vi "Send and Receive Message.vi"(4 "timeout (ms) [100]":i32=100, 6 "Wait for response [T]":bool=TRUE, 8 "error in (no error)":errorcluster, 9 "Data":variant, 10 "Command":string, 11 "RemoteControl in":refnum<class "RemoteControl.lvclass">) -> (0 "error out":errorcluster, 1 "Data out":variant, 2 "Command out":string, 3 "RemoteControl out":refnum<class "RemoteControl.lvclass">)   [LabVIEW 2019, in "RemoteControl.lvclass"]
uses:
  RemoteControl.lvclass
  <userlib>/_OpenG.lib/numeric/numeric.llb/Random Number Within Range - I32__ogtk.vi
  <vilib>/Utility/error.llb/Error Cluster From Error Code.vi
  <vilib>/ErrorRing/Error Ring.xnode
panel:
  out "Numeric":i32
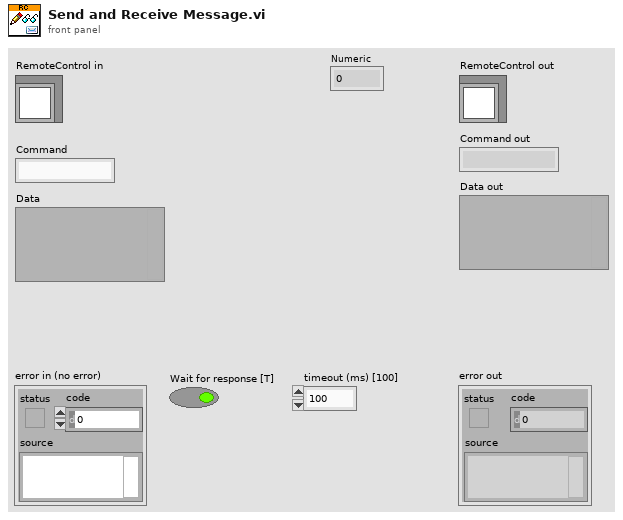
[diagram p1: front panel]
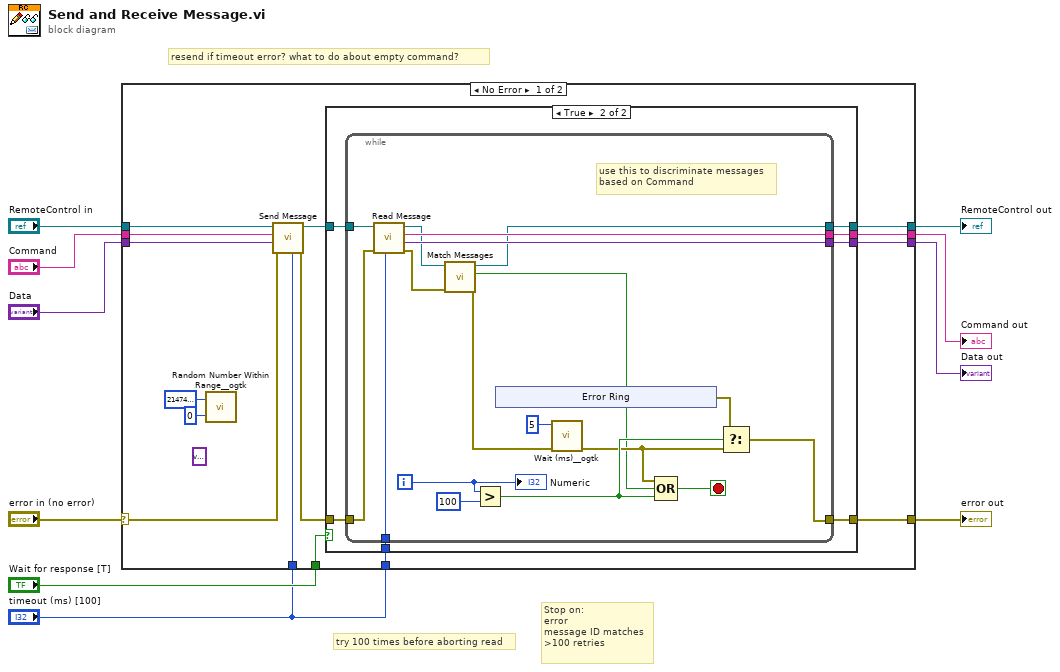
[diagram p0: block diagram]
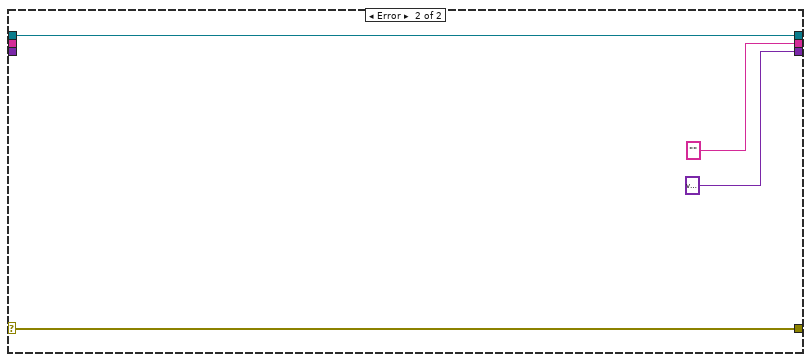
[diagram p3: hidden frame]
diagram:
  # "Stop on:\nerror\nmessage ID matches\n>100 retries"
  # "resend if timeout error? what to do about empty command?"
  # "try 100 times before aborting read"
  n1 = case shown="No Error" "error in (no error)" {
    selector: "error in (no error)" -> [w13 w60]
    tunnel: [w14 w60] -> w9
    tunnel: [w20 w59] -> w7
    tunnel: "RemoteControl in" -> [w22 w59]
    tunnel: "Wait for response [T]" -> [w25 _]
    tunnel: "timeout (ms) [100]" -> [w24 _]
    tunnel: "timeout (ms) [100]" -> [w21 _]
    tunnel: "Command" -> [w11 _]
    tunnel: "Data" -> [w19 _]
    tunnel: [w18 "" ("Command")] -> w2
    tunnel: [w17 variant ("Data")] -> w1
    frame No Error {
      (unwired) variant
      n2 = call-poly <userlib>:"Random Number Within Range__ogtk.vi"("High"=2147483647, "Low"=0) -> ()  [unwired: 3 in, 1 out]
      n3 = call-dynamic "Send Message.vi"("timeout in ms (100)"=w21, "error in (no error)"=w13, "Data"=w19, "Command"=w11, "RemoteControl in"=w22) -> ("error out"=w12:errorcluster, "RemoteControl out"=w23:refnum<class "RemoteControl.lvclass">)  [unwired: 4 in, 1 out]
      n4 = case shown="True" w25 {
        tunnel: w23 -> [w26 w34]
        tunnel: [w26 w33] -> w20
        tunnel: [_ w32] -> w18
        tunnel: [_ w31] -> w17
        tunnel: [w27 w30] -> w14
        tunnel: w12 -> [w27 w29]
        tunnel: w24 -> [_ w28]
        frame False {
        }
        frame True {
          n5 = while {
            tunnel: [w38] -> w32
            tunnel: [w51] -> w31
            tunnel: w28 -> [w47]
            tunnel: w29 -> [w50]
            tunnel: [w45] -> w30
            tunnel: w34 -> [w52]
            tunnel: [w35] -> w33
            i -> [w42]
            stop <- w48 stop-if-true
            # "use this to discriminate messages\nbased on Command"
            n6 = call-dynamic "Read Message.vi"("timeout in ms (100)"=w47, "error in (no error)"=w50, "RemoteControl in"=w52) -> ("error out"=w40:errorcluster, "Data"=w51:variant, "Command"=w38:string, "RemoteControl out"=w36:refnum<class "RemoteControl.lvclass">)  [unwired: 4 in, 1 out]
            n7 = call-dynamic "Match Messages.vi"("error in (no error)"=w40, "RemoteControl in"=w36) -> ("error out"=w39:errorcluster, "Match"=w37:bool, "RemoteControl out"=w35:refnum<class "RemoteControl.lvclass">)  [unwired: 7 in]
            n8 = Greater?(x=w42, y=100) -> (0:w46:bool)
            n9 = xnode "Error Ring"() -> ("error out"=w44:errorcluster)
            n10 = call <userlib>:"Wait (ms)__ogtk.vi"("error in (no error)"=w39, "milliseconds to wait"=u32 5) -> ("error out"=w41:errorcluster)  [unwired: 8 in, 1 out]
            n11 = Compound Arithmetic op=OR(w41, w37, w46) -> (w48:bool)
            n12 = Select(t=w44, s=w46, f=w41) -> (s? t:f=w45:errorcluster)
            "Numeric" <- w42
          }
        }
      }
    }
    frame Error {
    }
  }
  "error out" <- w9
  "RemoteControl out" <- w7
  "Command out" <- w2
  "Data out" <- w1
